vi "Lock-in frequency.vi"(8 "error in (no error)":errorcluster, 9 "read-only? (t)":bool=TRUE, 10 "set frequency (Hz)":dbl, 11 "VISA resource name":refnum<visa-resource-name>) -> (0 "error out":errorcluster, 2 "frequency (Hz)":dbl, 3 "VISA resource name out":refnum<visa-resource-name>)   [LabVIEW 2009, in "SR830.lvlib"]
doc: "Sets and/or reads the current frequency of the lock-in amplifier. Note: to set the frequency, the lock-in reference mode must first be set to internal."
uses:
  sr830/SR830.lvlib
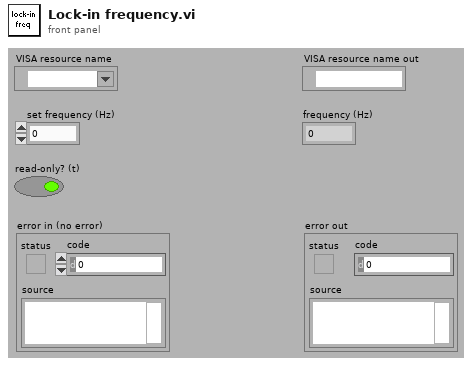
[diagram p1: front panel]
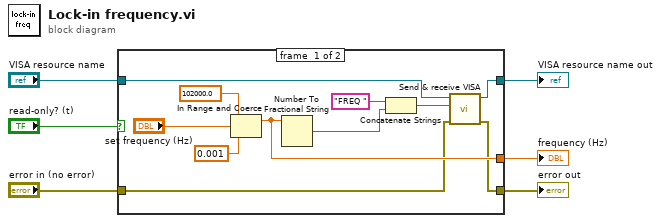
[diagram p0: block diagram]
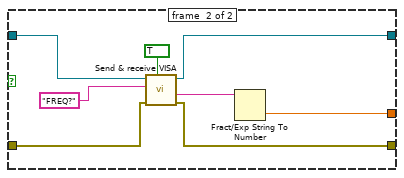
[diagram p2: hidden frame]
diagram:
  n1 = case shown="False" "read-only? (t)" {
    tunnel: [w12 w18] -> w6
    tunnel: "error in (no error)" -> [w11 w22]
    tunnel: [w10 w21] -> w3
    tunnel: "VISA resource name" -> [w9 w20]
    tunnel: [w8 w19] -> w1
    frame #0 {
      n2 = In Range and Coerce(upper limit=102000.0, x="set frequency (Hz)", lower limit=0.001) -> (coerced(x)=w12:dbl)  [unwired: 1 out]
      n3 = Number To Fractional String(number=w12) -> (F-format string=w13:string)  [unwired: 3 out]
      n4 = Concatenate Strings("FREQ " ("write buffer"), w13) -> (w14:string)
      n5 = call "Send & receive VISA.vi"("error in (no error)"=w11, "write buffer"=w14, "VISA resource name"=w9) -> ("error out"=w10:errorcluster, "VISA resource name out"=w8:refnum<visa-resource-name>)  [unwired: 2 in, 5 out]
    }
    frame #1 {
      n6 = call "Send & receive VISA.vi"("read? (f)"=TRUE, "error in (no error)"=w22, "write buffer"="FREQ?", "VISA resource name"=w20) -> ("error out"=w21:errorcluster, "read buffer"=w23:string, "VISA resource name out"=w19:refnum<visa-resource-name>)  [unwired: 1 in, 4 out]
      n7 = Fract/Exp String To Number(string=w23) -> (number=w18:dbl)  [unwired: 4 out]
    }
  }
  "frequency (Hz)" <- w6
  "error out" <- w3
  "VISA resource name out" <- w1
